vi "to_toml_string.vi"(8 "error in (no error)":errorcluster, 11 "Doc in":refnum<class "Doc.lvclass">) -> (0 "error out":errorcluster, 2 "toml_string":string, 3 "Doc out":refnum<class "Doc.lvclass">)   [LabVIEW 2020, in "toml_edit.lvlib" / "Doc.lvclass"]
uses:
  Doc.lvclass
  Doc.lvclass/Doc.ctl
  toml_edit.lvlib
  dragon_toml_64.dll
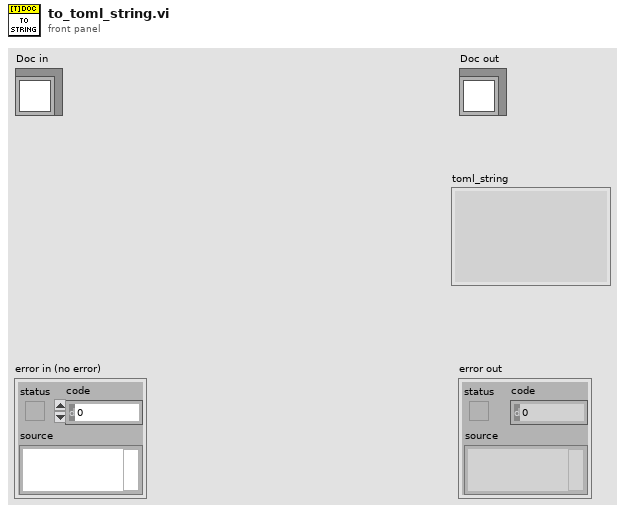
[diagram p1: front panel]
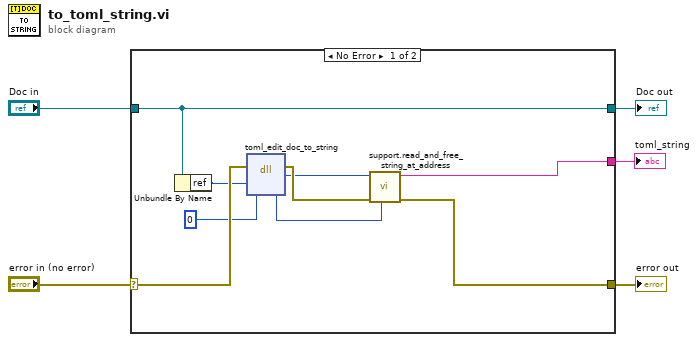
[diagram p0: block diagram]
diagram:
  n1 = case shown="No Error" "error in (no error)" {
    selector: "error in (no error)" -> [w14 w16]
    tunnel: [w10 w16] -> w4
    tunnel: [w13 w15] -> w2
    tunnel: "Doc in" -> [w13 w15]
    tunnel: [w8 _] -> w1
    frame No Error {
      n2 = Unbundle By Name(w13) -> ("ref"=w12:u64)
      n3 = dll-call lib="C:/projects/dragon-desktop/source/submodules/toml-edit-labview/lv_src/dragon_toml_*.dll" fn="toml_edit_doc_to_string"(error in=w14, "doc_ref"=w12, "string_length"=u32 0) -> (error out=w11:errorcluster, "table_names_ptr"=w9:u64, "string_length"=w6:u32)  [unwired: 3 in, 1 out]
      n4 = call "support.read_and_free_string_at_address.vi"("string_length"=w6, "error in (no error)"=w11, "string_ptr"=w9) -> ("error out"=w10:errorcluster, "string"=w8:string)  [unwired: 7 in]
    }
    frame Error {
    }
  }
  "error out" <- w4
  "Doc out" <- w2
  "toml_string" <- w1
